vi "G8CINuInt32Trace_v2_sub.vi"(0 "Macros":i32[](array[numeric]), 1 "bin time (ns)":i32=10000) -> (2 "error":bool, 3 "Trace Length":i32=46, 4 "G1-G8":sgl[](array[numeric])=[0.09877741, 0.10254161, 0.11935602, 0.14294545, 0.1540673, 0.14321436, 0.17901224, 0.16391604] format="%.2f")   [LabVIEW 2009]
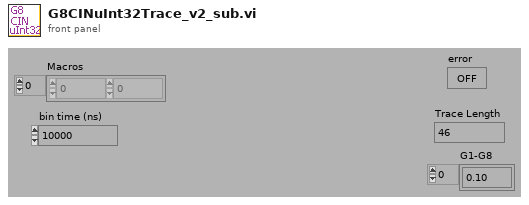
[diagram p1: front panel]
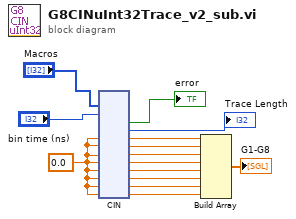
[diagram p0: block diagram]
diagram:
  w10 = sgl 0.0
  n1 = cin("Macros", "bin time (ns)", w10, w10, w10, w10, w10, w10, w10, w10) -> (→"error":bool, →"Trace Length":i32, w8:sgl, w7:sgl, w6:sgl, w5:sgl, w4:sgl, w3:sgl, w2:sgl, w1:sgl)  [unwired: 4 in]
  n2 = Build Array(w8, w7, w6, w5, w4, w3, w2, w1) -> (→"G1-G8":sgl[])
